vi "Script PD.vi"(6 "PD Cluster":refnum<vi>, 8 "error in":errorcluster, 9 "PD Control":refnum<vi>, 10 "Terminal Attributes":T1) -> (0 "error out":errorcluster)   [LabVIEW 2025, in "_Rescript.lvlib" / "Msg.lvlib" / "Msg.lvclass"]
uses:
  Msg.lvclass
  Terminal Attributes.ctl
  Attributes.ctl
  Msg.lvclass/Msg.ctl
  _Rescript.lvlib
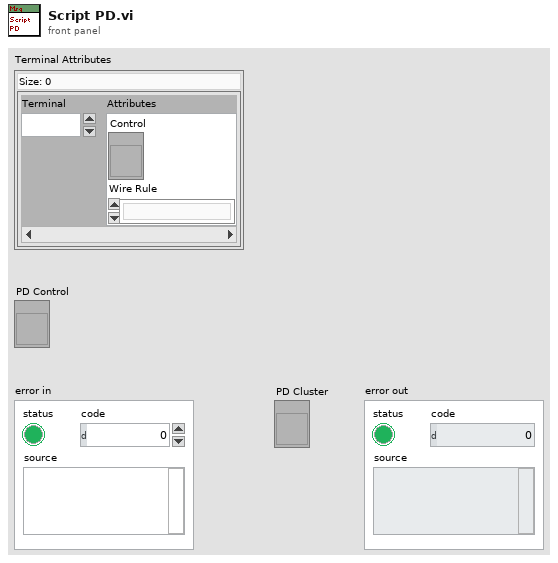
[diagram p1: front panel]
types:
  T1 = typedef "_Rescript.lvlib/Terminal Attributes.ctl" = map{i32, T2}
  T2 = typedef "_Rescript.lvlib/Attributes.ctl" = cluster{"Control":refnum<vi>, "Wire Rule":enum16{"Invalid Wire Rule", "Required", "Recommended", "Optional", "Dynamic Dispatch"}}
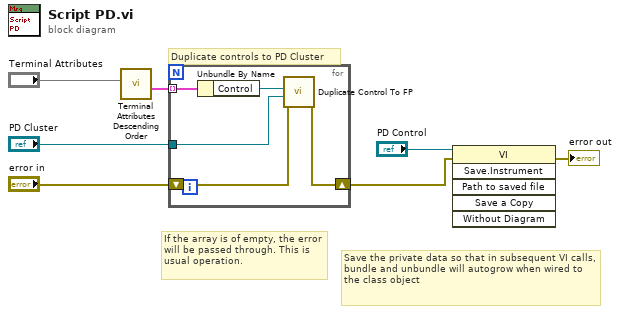
[diagram p0: block diagram]
diagram:
  # "If the array is of empty, the error will be passed through. This is usual operation."
  # "Duplicate controls to PD Cluster"
  # "Save the private data so that in subsequent VI calls, bundle and unbundle will autogrow when wired to the class object"
  n1 = call "Terminal Attributes Descending Order.vi"("Terminal Attributes"="Terminal Attributes") -> ("Attributes Descending Order"=w1:T2[])  [unwired: 9 in, 1 out]
  n2 = for {
    tunnel: "PD Cluster" -> [w12]
    shift-right: [w10] -> w4
    shift-left: "error in" -> [w11]
    tunnel: w1 -> [w9] mode=indexing
    n3 = Unbundle By Name(w9) -> ("Control"=w8:refnum<vi>)
    n4 = call "Duplicate Control To FP.vi"("error in"=w11, "Owner"=w12, "Control"=w8) -> ("error out"=w10:errorcluster)  [unwired: 8 in]
  }
  n5 = invoke class="VI" method="Save.Instrument"(reference="PD Control", error in=w4) -> (error out=→"error out":errorcluster)  [unwired: 4 in, 5 out]
